vi "Chamber control Feb_2018.vi"() -> ()   [LabVIEW 2014]
doc: "This template is for the Queued Message Handler design pattern.\n\nThe Event Handling Loop generates messages based on user interface actions.\n\nThe Message Handling Loop processes messages generated by the Event Handling Loop, or by other messages. The messages are string values, so new messages can be added easily to the Message Cases case structure in the Message Handling Loop. Each message cluster can also provide an optional value for Message Data, which is a variant that can be converted to whatever message-specific data is required."
uses:
  <vilib>/Analysis/baseanly.llb/Mean (DBL).vi
  <vilib>/Instr/_visa.llb/VISA Configure Serial Port (Instr).vi
  Environmental Chamber LabVIEW and Instruments/Drivers and Software/Keithley 2100 Series/Public/Configure/Configure 2 Wire Resistance.vi
  <vilib>/Utility/file.llb/Write To Spreadsheet File (string).vi
  <vilib>/Utility/file.llb/Read From Spreadsheet File (string).vi
  Environmental Chamber LabVIEW and Instruments/Drivers and Software/LabVIEW 8.2 Drivers/keithley_24xx/Keithley 24XX/Public/Data/Read (Single Point).vi
  Environmental Chamber LabVIEW and Instruments/Drivers and Software/keithley_6430/Keithley 6430/Public/Data/Read (Single Point).vi
  Environmental Chamber LabVIEW and Instruments/Drivers and Software/keithley_6430/Keithley 6430/Keithley 6430.lvlib
  Environmental Chamber LabVIEW and Instruments/Drivers and Software/Keithley 2100 Series/Keithley 2100 Series.lvlib
  Environmental Chamber LabVIEW and Instruments/Drivers and Software/keithley_24xx/Keithley 24XX/Keithley 24XX.lvlib
  <vilib>/Analysis/NI_AALBase.lvlib
panel:
  in  "K2420 Applied Voltage (V)":dbl=0.05
  in  "SYSTEM CONTROL":T1={"valve % open"=0.0, "Desired pressure"=0.0, "set Vapor sccm"=0.0, "set Gas sccm"=0.0, "Valve mode"=enum."% Open", "Pressure Mode"=enum."Abs. pressure", "analyte partial pressure"=23.8, "Actual"=0.0, "Read pressure (Torr)"=0.0, "Read vapor flow (sccm)"=0.0, "Read gas flow (sccm)"=0.0, "Save now"=FALSE, "Stop after seq."=TRUE, "Turbo pump\nauto on"=TRUE, "Integrate points"=0} caption="Pressure settings" {"Integrate points" min=0 max=100 step=1; "analyte partial pressure" min=0.0 max=100.0 step=5.0; "set Gas sccm" min=0 max=200 step=5; "set Vapor sccm" min=0 max=200 step=5; "Desired pressure" min=0.0 max=760.0 step=5.0; "valve % open" min=0.0 max=100.0 step=5.0 format="%#_2f"}
  in  "SAVE SAMPLE / ANALYTE NAMES":T2={"QCM1"="", "QCM2"="", "QCM3"="", "QCM4"="broken", "QCM5"="NOT WORKING", "QCM6"="", "SRS"="bareAu", "K-2420"="", "K-6430"="", "K-2100"="", "Gas"="NOT WORKING", "Vapor"="H2O", "Notes"=""} caption="Save samplffe names"
  in  "Clear all charts":bool
  out "K-6430":dbl(graph)
  out "K-2420":dbl(graph)
  out "File":path caption="DATA FILE"
  in  "Stop":bool
  out "QCM plot":T3(graph)
  out "K-2100":dbl(graph)
  out "State date/time":string caption="Program start time"
  out "J-KEM temp":dbl(graph)
  out "saving data?":bool
  out "pressure chart":dbl(graph)
  out "arduino qcm stack plot":T4(graph)
  in  "SEQUENCE":T5 {"preview" items=["pressure", "gas flow", "vapor flow", "bias"]}
  # "100"
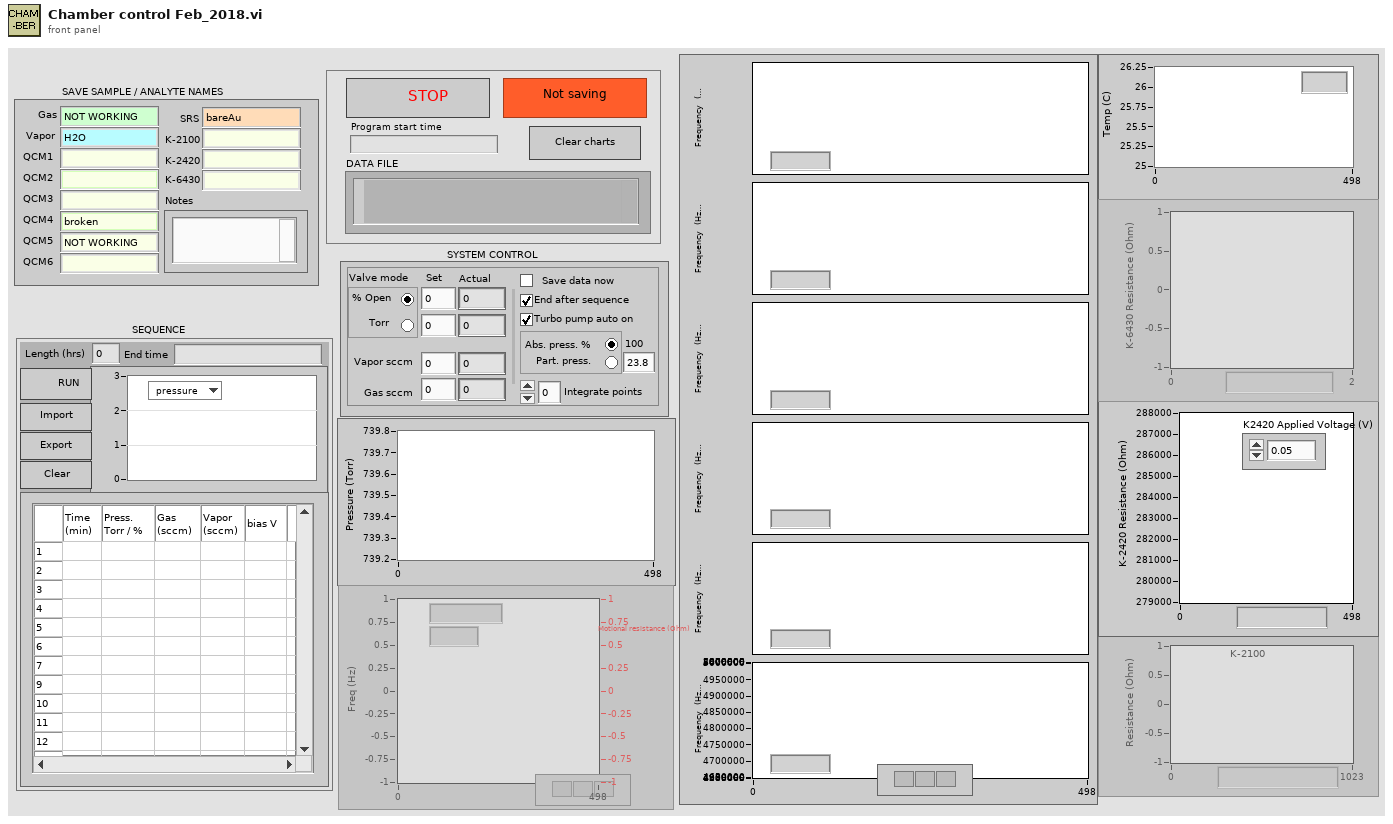
[diagram p1: front panel]
types:
  T1 = cluster{"valve % open":dbl, "Desired pressure":dbl, "set Vapor sccm":sgl, "set Gas sccm":sgl, "Valve mode":enum32{"% Open", "Torr "}, "Pressure Mode":enum32{"Abs. pressure", " Part. pressure"}, "analyte partial pressure":dbl, "Actual":dbl, "Read pressure (Torr)":dbl, "Read vapor flow (sccm)":dbl, "Read gas flow (sccm)":dbl, "Save now":bool, "Stop after seq.":bool, "Turbo pump\nauto on":bool, "Integrate points":i32}
  T2 = cluster{"QCM1":string, "QCM2":string, "QCM3":string, "QCM4":string, "QCM5":string, "QCM6":string, "SRS":string, "K-2420":string, "K-6430":string, "K-2100":string, "Gas":string, "Vapor":string, "Notes":string}
  T3 = cluster{"Frequency out":dbl, "Resistance out":dbl}
  T4 = cluster{"[0]":dbl, "[1]":dbl, "[2]":dbl, "[3]":dbl, "[4]":dbl, "[5]":dbl}
  T5 = cluster{"Run Sequence":bool, "User-defined\nsequence":string[][], "preview":u16, "Sequence\npreview":cluster{dbl[], dbl[]}[], "Save sequence":bool, "Clear sequence":bool, "Import sequence file":bool, "Length (hrs)":dbl, "End time":string}
  T6 = cluster{"Keithley 6430":bool, "J-KEM":bool, "Keithley 2420":bool, "Keithley 2100":bool, "SRS QCM":bool, "Pressure control":bool, "Arduino":bool}
  T7 = enum16{"open", "replace", "create", "open or create", "replace or create", "replace or create with confirmation"}
  T8 = cluster{"Arduino 1":refnum<visa-resource-name>, "Arduino 2":refnum<visa-resource-name>, "Arduino 3":refnum<visa-resource-name>, "Arduino 4":refnum<visa-resource-name>, "Arduino 5":refnum<visa-resource-name>, "Arduino 6":refnum<visa-resource-name>}
  T9 = enum8{"Enabled", "Disabled", "Disabled and Grayed Out"}
  T10 = cluster{"[0]":dbl, "[1]":dbl, "[2]":dbl, "[3]":dbl, "[4]":dbl, "[5]":dbl}[]
  T11 = cluster{"Frequency out":dbl, "Resistance out":dbl}[]
  T12 = cluster{"VISA resource name":refnum<visa-resource-name>, "error out":errorcluster, bool}
  T13 = cluster{"VISA resource name out":refnum<visa-resource-name>, "error out":errorcluster, bool}
  T14 = cluster{bool, "task out":refnum<k21>, "error out":errorcluster, "task out":refnum<k21>, "error out":errorcluster, "turbo pump":refnum<visa-resource-name>, "error out":errorcluster}
  T15 = cluster{bool, "task out":refnum<k21>, "error out":errorcluster, "task out":refnum<k21>, "error out":errorcluster, "VISA resource name out":refnum<visa-resource-name>, "error out":errorcluster}
  T16 = cluster{bool, "VISA resource name":refnum<visa-resource-name>, "error out":errorcluster}
  T17 = cluster{bool, "VISA resource name out":refnum<visa-resource-name>, "error out":errorcluster}
  T18 = cluster{bool, "VISA in":refnum<visa-resource-name>, "error out":errorcluster}
  T19 = cluster{bool, "VISA out":refnum<visa-resource-name>, "error out":errorcluster}
  T20 = cluster{"Arduino address":refnum<visa-resource-name>, "error in (no error)":errorcluster, "Arduino address 2":refnum<visa-resource-name>, "error in (no error) 2":errorcluster, "Arduino address 3":refnum<visa-resource-name>, "error in (no error) 3":errorcluster, "Arduino address 4":refnum<visa-resource-name>, "error in (no error) 4":errorcluster, "Arduino address 5":refnum<visa-resource-name>, "error in (no error) 5":errorcluster, "Arduino address 6":refnum<visa-resource-name>, "error in (no error) 6":errorcluster, "arduinos on?":bool}
  T21 = cluster{string[][], path, "data headers":string[]}
  T22 = cluster{"valve % open":dbl, "Desired pressure":dbl, "set Vapor sccm":sgl, "set Gas sccm":sgl, "Valve mode":enum32{"% Open", "Torr "}, "Pressure Mode":enum32{"Abs. pressure", " Part. pressure"}, "analyte partial pressure":dbl}
  T23 = cluster{"Boolean":bool, "VISA resource name out":refnum<visa-resource-name>, "error out":errorcluster}
  T24 = cluster{"Boolean":bool, "VISA out":refnum<visa-resource-name>, "error out":errorcluster}
  T25 = cluster{"Boolean":bool, "Arduino address":refnum<visa-resource-name>, "error in (no error)":errorcluster, "Arduino address 2":refnum<visa-resource-name>, "error in (no error) 2":errorcluster, "Arduino address 3":refnum<visa-resource-name>, "error in (no error) 3":errorcluster, "Arduino address 4":refnum<visa-resource-name>, "error in (no error) 4":errorcluster, "Arduino address 5":refnum<visa-resource-name>, "error in (no error) 5":errorcluster, "Arduino address 6":refnum<visa-resource-name>, "error in (no error) 6":errorcluster}
  T26 = cluster{"arduino addresses out":cluster{"Boolean":bool, "Arduino address":refnum<visa-resource-name>, "error in (no error)":errorcluster, "Arduino address 2":refnum<visa-resource-name>, "error in (no error) 2":errorcluster, "Arduino address 3":refnum<visa-resource-name>, "error in (no error) 3":errorcluster, "Arduino address 4":refnum<visa-resource-name>, "error in (no error) 4":errorcluster, "Arduino address 5":refnum<visa-resource-name>, "error in (no error) 5":errorcluster, "Arduino address 6":refnum<visa-resource-name>, "error in (no error) 6":errorcluster}, cluster{bool, "VISA resource name out":refnum<visa-resource-name>, "error out":errorcluster}, "Address out":cluster{"Boolean":bool, "VISA resource name out":refnum<visa-resource-name>, "error out":errorcluster}, cluster{bool, "VISA resource name out":refnum<visa-resource-name>, "error out":errorcluster}, cluster{bool, "VISA resource name out":refnum<visa-resource-name>, "error out":errorcluster}, "SRS address out":cluster{"Boolean":bool, "VISA out":refnum<visa-resource-name>, "error out":errorcluster}}
  T27 = cluster{"User-defined\nsequence":string[][], "Present (s)":dbl, "current  step # in":i32, "sequence end time in":timestamp}
  T28 = cluster{"current  step # in":i32, "sequence end time in":timestamp, "Boolean":bool}
  T29 = cluster{"press/RH/gas/vapor":cluster{"pressure":string, "RH":string, "gas flow":string, "vapor flow":string}, "Cluster":cluster{"Valve position (%)":dbl, "read pressure":dbl, "read vapor flow":dbl, "read gas flow":dbl}}
  T30 = cluster{"Boolean":bool, "task out":refnum<k21>, "error out":errorcluster, "task out":refnum<k21>, "error out":errorcluster, "VISA resource name out":refnum<visa-resource-name>, "error out":errorcluster}
  T31 = cluster{"pressure":string, "RH":string, "gas flow":string, "vapor flow":string}
  T32 = cluster{"Valve position (%)":dbl, "read pressure":dbl, "read vapor flow":dbl, "read gas flow":dbl}
  T33 = cluster{"[0]":string, "[1]":string, "[2]":string, "[3]":string, "[4]":string, "[5]":string}
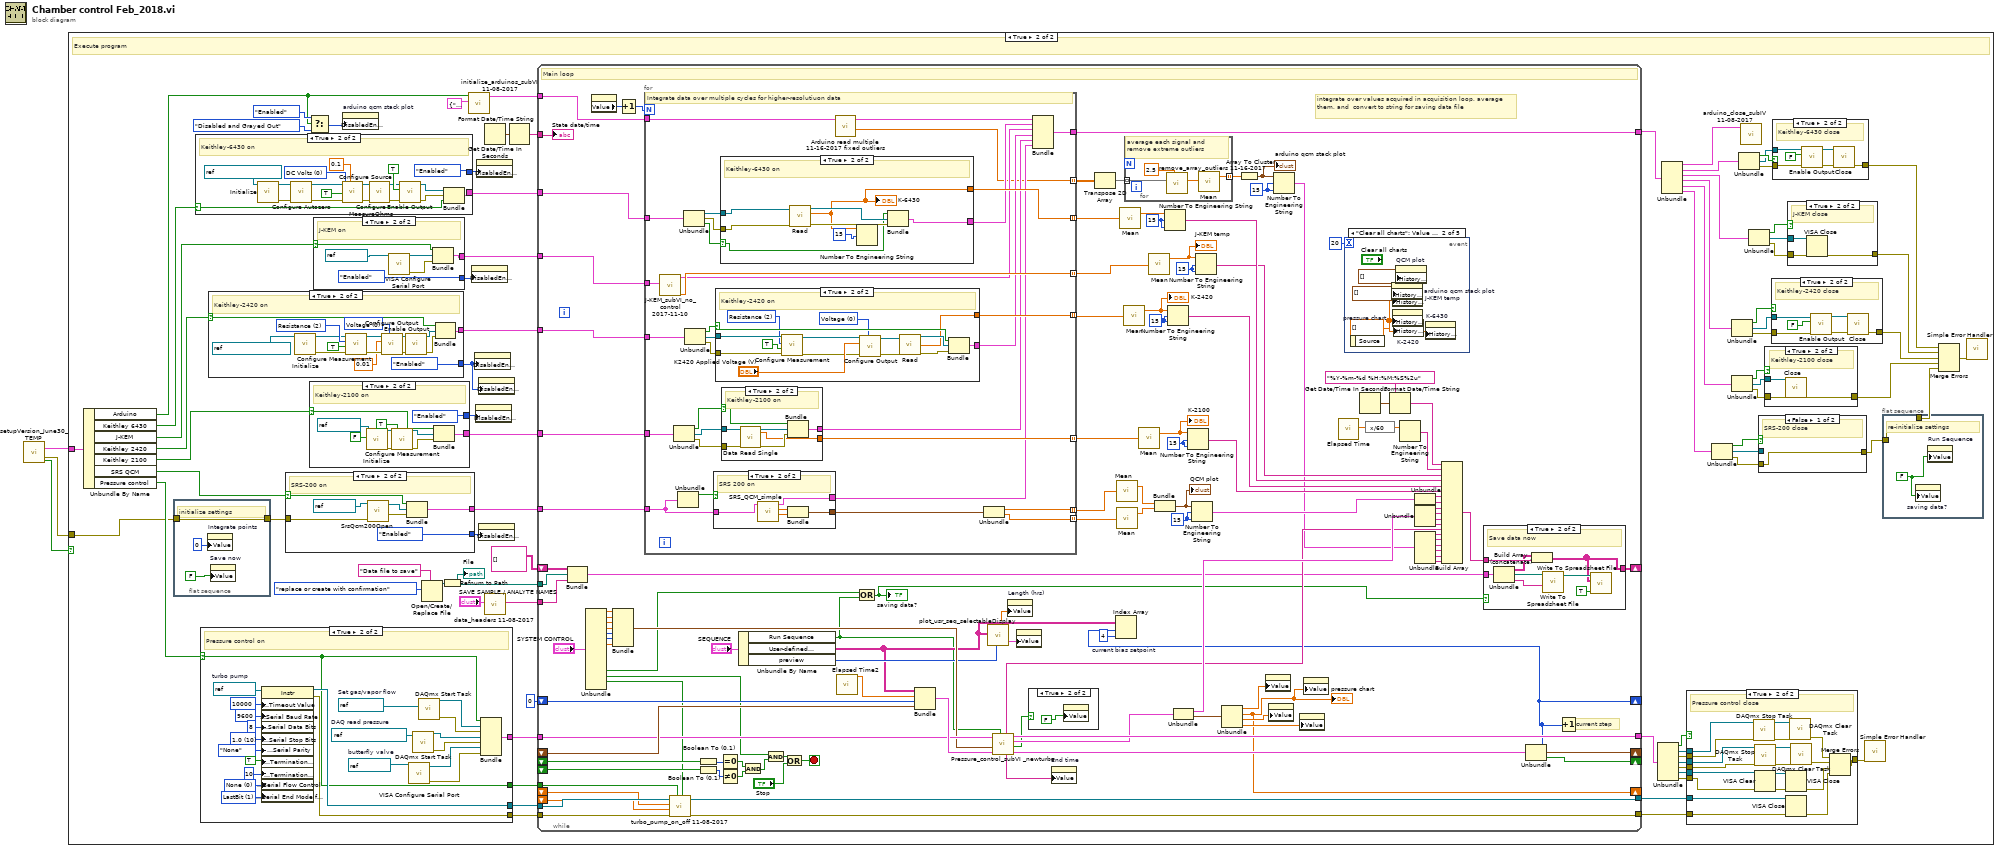
[diagram p0: block diagram]
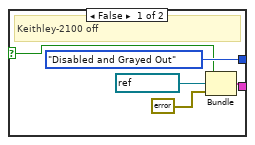
[diagram p4: hidden frame]
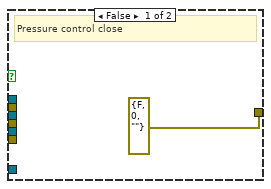
[diagram p5: hidden frame]
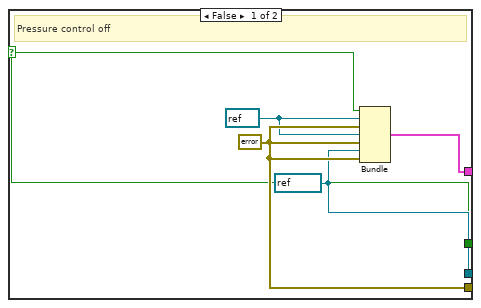
[diagram p6: hidden frame]
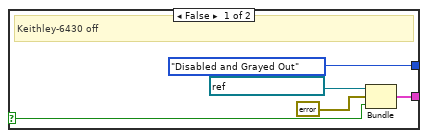
[diagram p8: hidden frame]
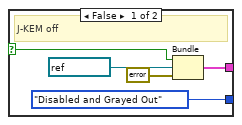
[diagram p10: hidden frame]
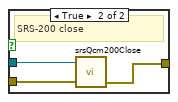
[diagram p11: hidden frame]
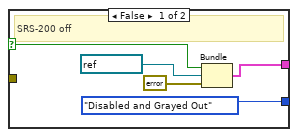
[diagram p12: hidden frame]
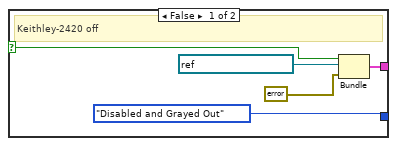
[diagram p14: hidden frame]
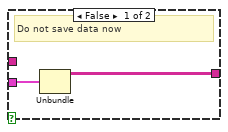
[diagram p15: hidden frame]
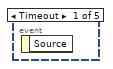
[diagram p16: hidden frame]
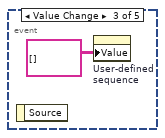
[diagram p17: hidden frame]
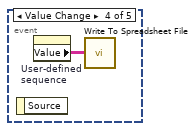
[diagram p18: hidden frame]
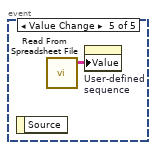
[diagram p19: hidden frame]
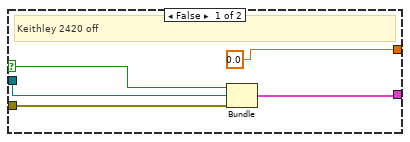
[diagram p20: hidden frame]
diagram:
  n1 = call "setupVersion_June30_TEMP.vi"() -> ("Instruments on/off"=w1:T6, "error IO"=w2:errorcluster, "OK"=w3:bool)  [unwired: 13 in]
  n2 = case shown="True" w3 {
    tunnel: w2 -> [_ w47]
    tunnel: w1 -> [_ w54]
    frame False {
      # "Cancel program"
    }
    frame True {
      # "Execute program"
      n3 = Unbundle By Name(w54) -> ("Arduino"=w26:bool, "Keithley 6430"=w53:bool, "J-KEM"=w52:bool, "Keithley 2420"=w51:bool, "Keithley 2100"=w50:bool, "SRS QCM"=w49:bool, "Pressure control"=w48:bool)
      n4 = flat-sequence {
        tunnel: [w85] -> w46
        tunnel: w47 -> [w85]
        frame #0 {
          # "initialize settings"
          n5 = property on="Integrate points" class="DigNum (strict)"("Value"=0) -> ()  [unwired: 2 in, 2 out]
          n6 = property on="Save now" class="Bool (strict)"("Value"=FALSE) -> ()  [unwired: 2 in, 2 out]
        }
      }
      n7 = case shown="True" w53 {
        selector: w53 -> [w163 w183]
        tunnel: [T9."Disabled and Grayed Out" ("Disabled") T9."Enabled" ("Disabled")] -> w32
        tunnel: [w162 w182] -> w30
        frame False {
          # "Keithley-6430 off"
          n8 = Bundle("VISA resource name"=refnum<visa-resource-name> "GPIB0::29::INSTR", "error out"=errorcluster {"status"=FALSE, "code"=0, "source"=""}, w163) -> (w162:T12)  [unwired: 1 in]
        }
        frame True {
          w170 = u16 0 items=["DC Volts", "DC Current"] ("Source Function (0: DC Volts)")
          # "Keithley-6430 on"
          n9 = call "Initialize.vi"("VISA resource name"=refnum<visa-resource-name> "GPIB2::19::INSTR") -> ("error out"=w176:errorcluster, "VISA resource name out"=w177:refnum<visa-resource-name>)  [unwired: 4 in, 5 out]
          n10 = call "Configure Autozero.vi"("error in (no error)"=w176, "VISA resource name"=w177) -> ("error out"=w173:errorcluster, "VISA resource name out"=w175:refnum<visa-resource-name>)  [unwired: 8 in]
          n11 = call "Configure Source.vi"("V-Source Level [V]"=0.1, "error in (no error)"=w173, "Auto Range (T:Enable)"=TRUE, "Source Function (0: DC Volts)"=w170, "VISA resource name"=w175) -> ("error out"=w172:errorcluster, "VISA resource name out"=w174:refnum<visa-resource-name>)  [unwired: 5 in]
          n12 = call "Configure MeasureOhms.vi"("error in (no error)"=w172, "VISA resource name"=w174) -> ("error out"=w181:errorcluster, "VISA resource name out"=w179:refnum<visa-resource-name>)  [unwired: 4 in, 4 out]
          n13 = call "Enable Output.vi"("error in (no error)"=w181, "Enable Output (F:Off)"=TRUE ("Output (F:Off)"), "VISA resource name"=w179) -> ("error out"=w168:errorcluster, "VISA resource name out"=w169:refnum<visa-resource-name>)  [unwired: 7 out]
          n14 = Bundle("VISA resource name out"=w169, "error out"=w168, w183) -> (w182:T13)  [unwired: 1 in]
        }
      }
      n15 = case shown="True" w48 {
        selector: w48 -> [w127 w133]
        tunnel: [w131 w134] -> w45
        tunnel: [w130 w132] -> w37
        tunnel: [w128 w135] -> w38
        tunnel: [w127 w133] -> w36
        frame False {
          w128 = refnum<visa-resource-name> refnum ("turbo pump")
          w129 = refnum<k21> refnum ("task out")
          w130 = errorcluster {"status"=FALSE, "code"=0, "source"=""} ("error out")
          # "Pressure control off"
          n16 = Bundle(w127, "task out"=w129, "error out"=w130, "task out"=w129, "error out"=w130, "turbo pump"=w128, "error out"=w130) -> (w131:T14)  [unwired: 1 in]
        }
        frame True {
          w139 = u16 1 items=["None", "LastBit", "TermChar"] ("Serial Settings:Serial End Mode for Reads")
          w137 = u16 0 items=["None", "XON/XOFF", "RTS/CTS", "XON/XOFF & RTS/CTS", "DTR/DSR", "XON/XOFF & DTR/DSR"] ("flow control (0:none)")
          w140 = u16 10 items=["1.0"=10, "1.5"=15, "2.0"=20] ("stop bits (10: 1 bit)")
          w136 = refnum<visa-resource-name> "COM7"  # turbo pump
          w152 = refnum<visa-resource-name> "COM5"  # butterfly valve
          w153 = refnum<k21> "Setflow"  # Set gas/vapor flow
          w154 = refnum<k21> "AllDaqReadings"  # DAQ read pressure
          # "Pressure control on"
          n17 = property class="Instr"(reference=w136, "General Settings:Timeout Value"=u32 10000 ("timeout (10sec)"), "Serial Settings:Serial Baud Rate"=u32 9600 ("baud rate (9600)"), "Serial Settings:Serial Data Bits"=u16 8 ("data bits (8)"), "Serial Settings:Serial Stop Bits"=w140, "Serial Settings:Serial Parity"=enum16{"None", "Odd", "Even", "Mark", "Space"}."None" ("parity (0:none)"), "Message Based Settings:Termination Character Enable"=TRUE ("Enable Termination\nChar (T)"), "Message Based Settings:Termination Character"=u8 10 ("termination char\n(0xA = '\\n' = LF)"), "Serial Settings:Serial Flow Control"=w137, "Serial Settings:Serial End Mode for Reads"=w139) -> (reference out=w135:refnum<visa-resource-name>, error out=w132:errorcluster)  [unwired: 1 in]
          n18 = call-poly "VISA Configure Serial Port"("VISA resource name"=w152) -> ("VISA resource name out"=w147:refnum<visa-resource-name>, "error out"=w146:errorcluster)  [unwired: 13 in]
          n19 = call <vilib>:"DAQmx Start Task.vi"("task/channels in"=w154) -> ("task out"=w149:refnum<k21>, "error out"=w148:errorcluster)  [unwired: 13 in]
          n20 = call <vilib>:"DAQmx Start Task.vi"("task/channels in"=w153) -> ("task out"=w151:refnum<k21>, "error out"=w150:errorcluster)  [unwired: 13 in]
          n21 = Bundle(w133, "task out"=w151, "error out"=w150, "task out"=w149, "error out"=w148, "VISA resource name out"=w147, "error out"=w146) -> (w134:T15)  [unwired: 1 in]
        }
      }
      n22 = case shown="True" w51 {
        selector: w51 -> [w226 w231]
        tunnel: [T9."Disabled and Grayed Out" ("Disabled") T9."Enabled" ("Disabled")] -> w11
        tunnel: [w224 w228] -> w29
        frame False {
          # "Keithley-2420 off"
          n23 = Bundle(w226, "VISA resource name"=refnum<visa-resource-name> "GPIB1::24::INSTR", "error out"=errorcluster {"status"=FALSE, "code"=0, "source"=""}) -> (w224:T16)  [unwired: 1 in]
        }
        frame True {
          w237 = u16 0 items=["Voltage", "Current"] ("Source Mode  (0: Voltage)")
          w242 = u16 2 items=["Volts", "Current", "Resistance"] ("Function (0: Volts)")
          # "Keithley-2420 on"
          n24 = call "Initialize.vi"("VISA resource name"=refnum<visa-resource-name> "GPIB1::24::INSTR") -> ("error out"=w232:errorcluster, "VISA resource name out"=w233:refnum<visa-resource-name>)  [unwired: 9 in]
          n25 = call "Configure Measurement.vi"("error in (no error)"=w232, "Enable Auto Range (T:Enable)"=TRUE, "Function (0: Volts)"=w242, "VISA resource name"=w233) -> ("error out"=w241:errorcluster, "VISA resource name out"=w240:refnum<visa-resource-name>)  [unwired: 6 in]
          n26 = call "Configure Output.vi"("Source Mode  (0: Voltage)"=w237, "error in (no error)"=w241, "Output Level (0)"=0.01 ("K2420 Applied Voltage (V) 2"), "VISA resource name"=w240) -> ("error out"=w239:errorcluster, "VISA resource name out"=w238:refnum<visa-resource-name>)  [unwired: 6 in]
          n27 = call "Enable Output.vi"("error in (no error)"=w239, "VISA resource name"=w238) -> ("error out"=w229:errorcluster, "VISA resource name out"=w230:refnum<visa-resource-name>)  [unwired: 8 in]
          n28 = Bundle(w231, "VISA resource name out"=w230, "error out"=w229) -> (w228:T17)  [unwired: 1 in]
        }
      }
      n29 = case shown="True" w49 {
        selector: w49 -> [w205 w211]
        tunnel: w46 -> [_ w214]
        tunnel: [T9."Disabled and Grayed Out" ("Disabled") T9."Enabled" ("Disabled")] -> w66
        tunnel: [w204 w210] -> w27
        frame False {
          # "SRS-200 off"
          n30 = Bundle(w205, "VISA in"=refnum<visa-resource-name> "COM6", "error out"=errorcluster {"status"=FALSE, "code"=0, "source"=""}) -> (w204:T18)  [unwired: 1 in]
        }
        frame True {
          # "SRS-200 on"
          n31 = call "SrsQcm200Open.vi"("error in"=w214, "VISA in"=refnum<visa-resource-name> "COM6") -> ("error out"=w209:errorcluster, "VISA out"=w212:refnum<visa-resource-name>)  [unwired: 3 in]
          n32 = Bundle(w211, "VISA out"=w212, "error out"=w209) -> (w210:T19)  [unwired: 1 in]
        }
      }
      n33 = Select(t=T9."Enabled" ("Disabled"), s=w26, f=T9."Disabled and Grayed Out" ("Disabled")) -> (s? t:f=w33:T9)
      n34 = case shown="True" w50 {
        selector: w50 -> [w95 w99]
        tunnel: [T9."Disabled and Grayed Out" ("Disabled") T9."Enabled" ("Disabled")] -> w63
        tunnel: [w92 w100] -> w28
        frame False {
          # "Keithley-2100 off"
          n35 = Bundle(w95, "VISA resource name out"=refnum<visa-resource-name> "K-2100", "error out"=errorcluster {"status"=FALSE, "code"=0, "source"=""}) -> (w92:T17)  [unwired: 1 in]
        }
        frame True {
          # "Keithley-2100 on"
          n36 = call "Initialize.vi"("VISA resource name"=refnum<visa-resource-name> "K-2100", "Reset? (T: Reset)"=FALSE) -> ("VISA resource name out"=w104:refnum<visa-resource-name>, "error out"=w103:errorcluster)  [unwired: 16 in]
          n37 = call-poly "Configure Measurement.vi"("VISA resource name"=w104, "error in (no error)"=w103, "Auto Range? (T: Auto)"=TRUE) -> ("VISA resource name out"=w98:refnum<visa-resource-name>, "error out"=w97:errorcluster)  [unwired: 15 in]
          n38 = Bundle(w99, "VISA resource name out"=w98, "error out"=w97) -> (w100:T17)  [unwired: 1 in]
        }
      }
      n39 = case shown="True" w52 {
        selector: w52 -> [w190 w196]
        tunnel: [w191 w197] -> w75
        tunnel: [T9."Disabled and Grayed Out" ("Disabled") T9."Enabled" ("Disabled")] -> w31
        frame False {
          # "J-KEM off"
          n40 = Bundle(w190, "VISA resource name"=refnum<visa-resource-name> "COM3", "error out"=errorcluster {"status"=FALSE, "code"=0, "source"=""}) -> (w191:T16)  [unwired: 1 in]
        }
        frame True {
          # "J-KEM on"
          n41 = call-poly "VISA Configure Serial Port"("VISA resource name"=refnum<visa-resource-name> "COM3") -> ("VISA resource name out"=w198:refnum<visa-resource-name>, "error out"=w195:errorcluster)  [unwired: 13 in]
          n42 = Bundle(w196, "VISA resource name out"=w198, "error out"=w195) -> (w197:T17)  [unwired: 1 in]
        }
      }
      n43 = property on="arduino qcm stack plot" class="WFChart (strict)"("DisabledEnum"=w33) -> ()  [unwired: 2 in, 2 out]
      n44 = Open/Create/Replace File(prompt="Data file to save", operation (0:open)=T7."replace or create with confirmation") -> (refnum out=w9:refnum<file>)  [unwired: 4 in, 2 out]
      n45 = Refnum to Path(1:w9) -> (0:w5:path)
      "File" <- w5
      n46 = call "initialize_arduinos_subVI 11-08-2017.vi"("arduino 1-6 addresses"=T8 {"Arduino 1"="COM25", "Arduino 2"="COM48", "Arduino 3"="COM21", "Arduino 4"="COM22", "Arduino 5"="COM23", "Arduino 6"="COM24"} ("Arduino COMs"), "arduinos on?"=w26) -> ("arduino addresses out"=w65:T20)  [unwired: 9 in]
      n47 = property on="J-KEM temp" class="WFChart (strict)"("DisabledEnum"=w31) -> ()  [unwired: 2 in, 2 out]
      n48 = property on="K-2420" class="WFChart (strict)"("DisabledEnum"=w11) -> ()  [unwired: 2 in, 2 out]
      n49 = property on="K-2100" class="WFChart (strict)"("DisabledEnum"=w63) -> ()  [unwired: 2 in, 2 out]
      n50 = property on="K-6430" class="WFChart (strict)"("DisabledEnum"=w32) -> ()  [unwired: 2 in, 2 out]
      n51 = property on="K2420 Applied Voltage (V)" class="DigNum (strict)"("DisabledEnum"=w11) -> ()  [unwired: 2 in, 2 out]
      n52 = property on="QCM plot" class="WFChart (strict)"("DisabledEnum"=w66) -> ()  [unwired: 2 in, 2 out]
      n53 = call "data_headers 11-08-2017.vi"("Sample names"="SAVE SAMPLE / ANALYTE NAMES") -> ("data headers"=w4:string[])  [unwired: 10 in]
      n54 = Get Date/Time In Seconds() -> (seconds since 1Jan1904=w12:timestamp)
      n55 = Format Date/Time String(seconds (now)=w12) -> (date/time string=w62:string)  [unwired: 2 in]
      n56 = while {
        tunnel: w75 -> [w363]
        tunnel: w5 -> [w250]
        tunnel: w65 -> [w316]
        tunnel: w62 -> [w345]
        tunnel: w45 -> [w332]
        shift-right: [w312] -> _
        shift-left: 0 ("1st step") -> [w337]
        shift-right: [w342] -> _
        shift-left: _ -> [w340]
        shift-right: [w341] -> _
        shift-left: _ -> [w339]
        shift-left: _ -> [w338]
        tunnel: [w336] -> w58
        tunnel: w38 -> [w331]
        tunnel: w37 -> [w330]
        tunnel: w36 -> [w315]
        tunnel: [w328] -> w35
        tunnel: [w329] -> w34
        tunnel: w30 -> [w320]
        tunnel: w29 -> [w319]
        tunnel: w28 -> [w318]
        tunnel: w27 -> [w317]
        shift-right: [w256] -> _
        shift-left: _ -> [w314]
        shift-left: _ -> [w313]
        tunnel: [w288] -> w19
        shift-right: [w253] -> _
        shift-left: string[][] [] -> [w251]
        tunnel: w4 -> [w249]
        stop <- w351 stop-if-true
        w280 = i16 15 ("width (-)")
        w281 = i16 15 ("width (-)")
        w282 = i16 15 ("width (-)")
        w283 = i16 15 ("width (-)")
        w284 = i16 15 ("width (-)")
        w285 = i16 15 ("width (-)")
        # "current step"
        # "integrate over values acquired in acquisition loop, average them, and  convert to string for saving data file"
        # "Main loop"
        n57 = Bundle(w251, w250, "data headers"=w249) -> (w248:T21)  [unwired: 1 in]
        n58 = Unbundle("SYSTEM CONTROL") -> ("valve % open"=w273:dbl, "Desired pressure"=w272:dbl, "set Vapor sccm"=w271:sgl, "set Gas sccm"=w270:sgl, "Valve mode"=w269:enum32{"% Open", "Torr "}, "Pressure Mode"=w268:enum32{"Abs. pressure", " Part. pressure"}, "analyte partial pressure"=w267:dbl, "Save now"=w259:bool, "Stop after seq."=w258:bool, "Turbo pump\nauto on"=w257:bool)  [unwired: 5 out]
        n59 = property on="Integrate points" class="DigNum (strict)"() -> ("Value"=w245:i32)  [unwired: 2 in, 2 out]
        n60 = Bundle("valve % open"=w273, "Desired pressure"=w272, "set Vapor sccm"=w271, "set Gas sccm"=w270, "Valve mode"=w269, "Pressure Mode"=w268, "analyte partial pressure"=w267) -> (w274:T22)  [unwired: 1 in]
        n61 = Increment(x=w245) -> (x+1=w287:i32)
        n62 = for {
          N: w287 -> [_]
          tunnel: w320 -> [w414]
          tunnel: w319 -> [w411]
          tunnel: w318 -> [w407]
          tunnel: w317 -> [w388]
          tunnel: w316 -> [w387]
          tunnel: w363 -> [w415]
          tunnel: [w402] -> w307 mode=indexing
          tunnel: [w401] -> w302 mode=indexing
          tunnel: [w400] -> w305 mode=indexing
          tunnel: [w399] -> w301 mode=indexing
          tunnel: [w397] -> w299 mode=indexing
          tunnel: [w396] -> w298 mode=indexing
          tunnel: [w386] -> w293 mode=indexing
          tunnel: [w390] -> w288
          # "Integrate data over multiple cycles for higher-resolutiuon data"
          n63 = call "J-KEM_subVI_no_control 2017-11-10.vi"("Address in"=w415) -> ("Temp (C)"=w400:dbl, "Address out"=w394:T23)  [unwired: 9 in]
          n64 = Unbundle(w407) -> (w406:bool, "VISA resource name out"=w405:refnum<visa-resource-name>, "error out"=w404:errorcluster)
          n65 = Unbundle(w388) -> (w389:bool)  [unwired: 2 out]
          n66 = Unbundle(w414) -> ("VISA resource name out"=w413:refnum<visa-resource-name>, "error out"=w403:errorcluster, w412:bool)
          n67 = Unbundle(w411) -> (w410:bool, "VISA resource name out"=w409:refnum<visa-resource-name>, "error out"=w408:errorcluster)
          n68 = case "SRS QCM" shown="True" w389 {
            tunnel: [w461 w467] -> w391
            tunnel: [T3 {"Frequency out"=0.0, "Resistance out"=0.0} ("freq, MR") w464] -> w398
            tunnel: w388 -> [w461 w463]
            frame False {
              # "SRS QCM off"
            }
            frame True {
              # "SRS 200 on"
              n69 = call "SRS_QCM_simple.vi"("SRS address in"=w463) -> ("Resistance out"=w466:dbl, "Frequency out"=w465:dbl, "SRS address out"=w467:T24)  [unwired: 8 in]
              n70 = Bundle("Frequency out"=w465, "Resistance out"=w466) -> (w464:T3)  [unwired: 1 in]
            }
          }
          n71 = case shown="True" w410 {
            selector: w410 -> [w420 w435]
            tunnel: [w417 w434] -> w393
            tunnel: w409 -> [w419 w427]
            tunnel: w408 -> [w418 w425]
            tunnel: [sgl 0.0 ("Resistance") w422] -> w401
            frame False {
              # "Keithley 2420 off"
              n72 = Bundle(w420, "VISA resource name out"=w419, "error out"=w418) -> (w417:T17)  [unwired: 1 in]
            }
            frame True {
              w423 = u16 2 items=["Volts", "Current", "Resistance"] ("Function (0: Volts)")
              w431 = u16 0 items=["Voltage", "Current"] ("Source Mode  (0: Voltage)")
              # "Keithley-2420 on"
              n73 = call "Configure Measurement.vi"("error in (no error)"=w425, "Enable Auto Range (T:Enable)"=TRUE, "Function (0: Volts)"=w423, "VISA resource name"=w427) -> ("error out"=w424:errorcluster, "VISA resource name out"=w426:refnum<visa-resource-name>)  [unwired: 6 in]
              n74 = call "Configure Output.vi"("Source Mode  (0: Voltage)"=w431, "error in (no error)"=w424, "Output Level (0)"="K2420 Applied Voltage (V)", "VISA resource name"=w426) -> ("error out"=w429:errorcluster, "VISA resource name out"=w430:refnum<visa-resource-name>)  [unwired: 6 in]
              n75 = call-poly "Read.vi"("VISA resource name"=w430, "error in (no error)"=w429) -> ("VISA resource name out"=w433:refnum<visa-resource-name>, "Resistance"=w422:sgl, "error out"=w432:errorcluster)  [unwired: 7 in, 4 out]
              n76 = Bundle(w435, "VISA resource name out"=w433, "error out"=w432) -> (w434:T17)  [unwired: 1 in]
            }
          }
          n77 = case "Keithley 6430" shown="True" w412 {
            selector: w412 -> [w452 w455]
            tunnel: w413 -> [w451 w457]
            tunnel: [w450 w454] -> w395
            tunnel: w403 -> [w449 w456]
            tunnel: [0.0 ("K6340 Bias (V)") w453] -> w402
            frame False {
              # "Keithley-6430 off"
              n78 = Bundle(w452, "VISA resource name out"=w451, "error out"=w449) -> (w450:T17)  [unwired: 1 in]
            }
            frame True {
              # "Keithley-6430 on"
              n79 = call-poly "Read.vi"("error in (no error)"=w456, "VISA resource name"=w457) -> ("error out"=w458:errorcluster, "Measurement"=w453:dbl, "VISA resource name out"=w459:refnum<visa-resource-name>)  [unwired: 1 in, 6 out]
              "K-6430" <- w453
              n80 = Number To Engineering String(3:i16 15 ("width (-)"), 4:w453) -> ()  [unwired: 2 in, 1 out]
              n81 = Bundle(w455, "VISA resource name out"=w459, "error out"=w458) -> (w454:T17)  [unwired: 1 in]
            }
          }
          n82 = case shown="True" w406 {
            selector: w406 -> [w440 w445]
            tunnel: w405 -> [w438 w447]
            tunnel: w404 -> [w439 w446]
            tunnel: [w437 w442] -> w392
            tunnel: [0.0 ("Measurement") w441] -> w399
            frame False {
              # "Keithley-2100 off"
              n83 = Bundle(w440, "VISA resource name out"=w438, "error out"=w439) -> (w437:T17)  [unwired: 1 in]
            }
            frame True {
              # "Keithley-2100 on"
              n84 = call "Data Read Single.vi"("VISA resource name"=w447, "error in (no error)"=w446) -> ("VISA resource name out"=w444:refnum<visa-resource-name>, "Measurement"=w441:dbl, "error out"=w443:errorcluster)  [unwired: 15 in]
              n85 = Bundle(w445, "VISA resource name out"=w444, "error out"=w443) -> (w442:T17)  [unwired: 1 in]
            }
          }
          n86 = call "Arduino read multiple 11-16-2017 fixed outliers.vi"("arduino addresses in"=w387) -> ("freq out"=w386:dbl[], "arduino addresses out"=w385:T25)  [unwired: 8 in]
          n87 = Unbundle(w398) -> ("Frequency out"=w397:dbl, "Resistance out"=w396:dbl)
          n88 = Bundle("arduino addresses out"=w385, w395, "Address out"=w394, w393, w392, "SRS address out"=w391) -> (w390:T26)  [unwired: 1 in]
        }
        n89 = call "turbo_pump_on_off 11-08-2017.vi"("Turbo pump\nauto on"=w257, "pressure control on?"=w315, "error in (no error)"=w330, "read pressure"=w313, "read pressure 2"=w314, "VISA Refnum in"=w331) -> ("error out"=w329:errorcluster, "VISA Refnum out"=w328:refnum<visa-resource-name>)  [unwired: 4 in]
        n90 = Boolean To (0,1)(Boolean=w339) -> (0, 1=w355:i16)
        n91 = Boolean To (0,1)(Boolean=w338) -> (0, 1=w354:i16)
        n92 = Equal To 0?(x=w355) -> (x = 0?=w352:bool)
        n93 = Not Equal To 0?(x=w354) -> (x != 0?=w353:bool)
        n94 = Unbundle By Name("SEQUENCE") -> ("Run Sequence"=w261:bool, "User-defined\nsequence"=w264:string[][], "preview"=w265:u16)
        n95 = And(x=w352, y=w353) -> (x .and. y?=w350:bool)
        n96 = And(x=w258, y=w350) -> (x .and. y?=w349:bool)
        n97 = Or(x=w349, y="Stop") -> (x .or. y?=w351:bool)
        n98 = call "Elapsed Time2"() -> ("Present (s)"=w279:dbl)  [unwired: 12 in, 7 out]
        n99 = Or(x=w259, y=w261) -> (x .or. y?=w252:bool)
        "saving data?" <- w252
        n100 = Bundle("User-defined\nsequence"=w264, "Present (s)"=w279, "current  step # in"=w337, "sequence end time in"=w340) -> (w344:T27)  [unwired: 1 in]
        n101 = call "plot_usr_seq_selectableDisplay.vi"("Display"=w265, "User-defined sequence"=w264) -> ("Sequence Preview"=w263:cluster{dbl[], dbl[]}[], "seq length (hours)"=w244:dbl)  [unwired: 8 in]
        n102 = call "Pressure_control_subVI _newturbo.vi"("Run Sequence"=w261, "user sequence, present (s) in, current step in, seq time in"=w344, "pressure parameters in"=w274, "pressure control on?/daq IDs/errors"=w332) -> ("current step # out, shift register time out, seq button on?"=w343:T28, "sequence over? USE THIS TO REINITIALIZE RUN SEQUENCE BUTTON SO PROGRAM ENDS"=w262:bool, "save press/RH/gasflow/vaporflow - read valve position/pressure/vaporflow/gasflow"=w335:T29, "pressure control on?/daq IDs/errors out"=w336:T30, "sequence end date/time string"=w255:string, "pressure_setpoint"=w333:string)  [unwired: 2 in]
        n103 = property on="Length (hrs)" class="DigNum (strict)"("Value"=w244) -> ()  [unwired: 2 in, 2 out]
        n104 = property on="Sequence\npreview" class="XYGraph (strict)"("Value"=w263) -> ()  [unwired: 2 in, 2 out]
        n105 = case shown="True" w262 {
          frame False {
          }
          frame True {
            n106 = property on="Run Sequence" class="Bool (strict)"("Value"=FALSE ("Run Sequence")) -> ()  [unwired: 2 in, 2 out]
          }
        }
        n107 = property on="End time" class="Str"("Value"=w255) -> ()  [unwired: 2 in, 2 out]
        n108 = Transpose 2D Array(2D array=w293) -> (transposed array=w292:dbl[][])
        n109 = call-poly <vilib>:"Mean.vi"("X"=w299) -> ("mean"=w297:dbl)  [unwired: 1 out]
        n110 = call-poly <vilib>:"Mean.vi"("X"=w298) -> ("mean"=w296:dbl)  [unwired: 1 out]
        n111 = call-poly <vilib>:"Mean.vi"("X"=w307) -> ("mean"=w309:dbl)  [unwired: 1 out]
        n112 = call-poly <vilib>:"Mean.vi"("X"=w302) -> ("mean"=w247:dbl)  [unwired: 1 out]
        "K-2420" <- w247
        n113 = for {
          tunnel: w292 -> [w383] mode=indexing
          tunnel: [w384] -> w291 mode=indexing
          # "average each signal and remove extreme outliers"
          n114 = call "remove_array_outliers 11-16-2017.vi"("n standard devs to filter"=2.5, "input array"=w383) -> ("filtered array out"=w382:dbl[])  [unwired: 9 in]
          n115 = call-poly <vilib>:"Mean.vi"("X"=w382) -> ("mean"=w384:dbl)  [unwired: 1 out]
        }
        n116 = call-poly <vilib>:"Mean.vi"("X"=w301) -> ("mean"=w246:dbl)  [unwired: 1 out]
        "K-2100" <- w246
        n117 = call-poly <vilib>:"Mean.vi"("X"=w305) -> ("mean"=w303:dbl)  [unwired: 1 out]
        "J-KEM temp" <- w303
        n118 = Bundle("mean"=w297, "mean"=w296) -> (w295:cluster{"mean":dbl, "mean":dbl})  [unwired: 1 in]
        "QCM plot" <- w295
        n119 = Number To Engineering String(2:w285, 3:w285, 4:w309) -> (0:w308:string)  [unwired: 1 in]
        n120 = Number To Engineering String(2:w283, 3:w283, 4:w247) -> (0:w306:string)  [unwired: 1 in]
        n121 = Unbundle(w335) -> ("press/RH/gas/vapor"=w334:T31, "Cluster"=w278:T32)
        n122 = Number To Engineering String(2:w282, 3:w282, 4:w246) -> (0:w300:string)  [unwired: 1 in]
        n123 = Number To Engineering String(2:w280, 3:w280, 4:w295) -> (0:w294:cluster{"mean":string, "mean":string})  [unwired: 1 in]
        n124 = Number To Engineering String(2:w284, 3:w284, 4:w303) -> (0:w304:string)  [unwired: 1 in]
        n125 = Unbundle(w278) -> ("Valve position (%)"=w277:dbl, "read pressure"=w256:dbl, "read vapor flow"=w276:dbl, "read gas flow"=w275:dbl)
        "pressure chart" <- w256
        n126 = Array To Cluster(array=w291) -> (cluster=w290:T4)
        "arduino qcm stack plot" <- w290
        n127 = property on="Actual" class="DigNum (strict)"("Value"=w277) -> ()  [unwired: 2 in, 2 out]
        n128 = property on="Read vapor flow (sccm)" class="DigNum (strict)"("Value"=w276) -> ()  [unwired: 2 in, 2 out]
        n129 = Number To Engineering String(2:w281, 3:w281, 4:w290) -> (0:w289:T33)  [unwired: 1 in]
        n130 = property on="Read gas flow (sccm)" class="DigNum (strict)"("Value"=w275) -> ()  [unwired: 2 in, 2 out]
        n131 = property on="Read pressure (Torr)" class="DigNum (strict)"("Value"=w256) -> ()  [unwired: 2 in, 2 out]
        n132 = call "Elapsed Time"() -> ("Elapsed Time (s)"=w310:dbl)  [unwired: 12 in, 7 out]
        n133 = event shown="[1] \"Clear all charts\": Value Change" {
          selector: _ -> [_ _ _ _ _]
          dyn-events: _ -> [_ _ _ _ _]
          timeout: 20 -> [_ _ _ _ _]
          event Timeout {
            n134 = event-data() -> ()  [unwired: 1 in, 1 out]
          }
          event "Clear all charts": Value Change {
            w375 = dbl[] [] ("History Data")
            n135 = event-data() -> ()  [unwired: 1 in, 1 out]
            n136 = property on="arduino qcm stack plot" class="WFChart (strict)"("History Data"=T10 []) -> ()  [unwired: 2 in, 2 out]
            n137 = property on="J-KEM temp" class="WFChart (strict)"("History Data"=w375) -> ()  [unwired: 2 in, 2 out]
            n138 = property on="pressure chart" class="WFChart (strict)"("History Data"=w375) -> ()  [unwired: 2 in, 2 out]
            n139 = property on="K-2420" class="WFChart (strict)"("History Data"=w375) -> ()  [unwired: 2 in, 2 out]
            n140 = property on="QCM plot" class="WFChart (strict)"("History Data"=T11 []) -> ()  [unwired: 2 in, 2 out]
            n141 = property on="K-6430" class="WFChart (strict)"("History Data"=w375) -> ()  [unwired: 2 in, 2 out]
          }
          event "SEQUENCE.Clear sequence": Value Change {
            n142 = event-data() -> ()  [unwired: 1 in, 1 out]
            n143 = property on="User-defined\nsequence" class="Tbl (strict)"("Value"=string[][] []) -> ()  [unwired: 2 in, 2 out]
          }
          event "SEQUENCE.Save sequence": Value Change {
            n144 = event-data() -> ()  [unwired: 1 in, 1 out]
            n145 = property on="User-defined\nsequence" class="Tbl (strict)"() -> ("Value"=w379:string[][])  [unwired: 2 in, 2 out]
            n146 = call-poly <vilib>:"Write To Spreadsheet File.vi"("2D data"=w379) -> ()  [unwired: 7 in, 1 out]
          }
          event "SEQUENCE.Import sequence file": Value Change {
            n147 = event-data() -> ()  [unwired: 1 in, 1 out]
            n148 = call-poly <vilib>:"Read From Spreadsheet File.vi"() -> ("all rows"=w380:string[][])  [unwired: 7 in, 4 out]
            n149 = property on="User-defined\nsequence" class="Tbl (strict)"("Value"=w380) -> ()  [unwired: 2 in, 2 out]
          }
        }
        n150 = Get Date/Time In Seconds() -> (seconds since 1Jan1904=w364:timestamp)
        n151 = expression code="x/60"(w310) -> (w311:dbl)
        n152 = Format Date/Time String(time format string (%c)="%Y-%m-%d %H:%M:%S%2u", seconds (now)=w364) -> (date/time string=w360:string)  [unwired: 1 in]
        n153 = Number To Engineering String ("elapsed time (min)")(4:w311) -> (0:w346:string)  [unwired: 3 in]
        n154 = Unbundle(w294) -> ("mean"=w347:string, "mean"=w361:string)
        n155 = Unbundle(w334) -> ("pressure"=w359:string, "RH"=w358:string, "gas flow"=w357:string, "vapor flow"=w356:string)
        n156 = Unbundle(w289) -> ("[0]"=w326:string, "[1]"=w325:string, "[2]"=w324:string, "[3]"=w323:string, "[4]"=w322:string, "[5]"=w321:string)
        n157 = Build Array(w360, w346, w304, w308, w306, w300, w347, w361, w359, w358, w357, w356, w333, w326, w325, w324, w323, w322, w321) -> (w254:string[])
        n158 = case shown="True" w252 {
          tunnel: w254 -> [_ w374]
          tunnel: [w365 w371] -> w253
          tunnel: w248 -> [w366 w370]
          frame False {
            # "Do not save data now"
            n159 = Unbundle(w366) -> (w365:string[][])  [unwired: 2 out]
          }
          frame True {
            # "Save data now"
            n160 = Unbundle(w370) -> (w369:string[][], w368:path, "data headers"=w367:string[])
            n161 = Build Array (concatenate)(w369, w374) -> (w371:string[][])
            n162 = call-poly <vilib>:"Write To Spreadsheet File.vi"("1D data"=w367, "file path (dialog if empty)"=w368) -> ("new file path (Not A Path if cancelled)"=w372:path)  [unwired: 6 in]
            n163 = call-poly <vilib>:"Write To Spreadsheet File.vi"("append to file? (new file:F)"=TRUE, "2D data"=w371, "file path (dialog if empty)"=w372) -> ()  [unwired: 5 in, 1 out]
          }
        }
        n164 = Unbundle(w343) -> ("current  step # in"=w312:i32, "sequence end time in"=w342:timestamp, "Boolean"=w341:bool)
        n165 = Index Array "current bias setpoint"(array=w264, index (row)=w312, index (col)=4 ("disabled index (col)")) -> ()  [unwired: 1 out]
        n166 = Increment(x=w312) -> ()  [unwired: 1 out]
        "State date/time" <- w345
      }
      n167 = Unbundle(w58) -> ("Boolean"=w57:bool, "task out"=w44:refnum<k21>, "error out"=w43:errorcluster, "task out"=w42:refnum<k21>, "error out"=w41:errorcluster, "VISA resource name out"=w40:refnum<visa-resource-name>, "error out"=w39:errorcluster)
      n168 = Unbundle(w19) -> ("arduino addresses out"=w18:T25, w17:T17, "Address out"=w16:T23, w15:T17, w14:T17, "SRS address out"=w13:T24)
      n169 = case shown="True" w57 {
        tunnel: [errorcluster {"status"=FALSE, "code"=0, "source"=""} ("error out") w118] -> w61
        tunnel: w44 -> [_ w117]
        tunnel: w43 -> [_ w116]
        tunnel: w42 -> [_ w115]
        tunnel: w41 -> [_ w112]
        tunnel: w40 -> [_ w113]
        tunnel: w39 -> [_ w114]
        tunnel: w35 -> [_ w109]
        tunnel: w34 -> [_ w108]
        frame False {
          # "Pressure control close"
        }
        frame True {
          # "Pressure control close"
          n170 = call <vilib>:"DAQmx Stop Task.vi"("task/channels in"=w117, "error in"=w116) -> ("task out"=w124:refnum<k21>, "error out"=w123:errorcluster)  [unwired: 12 in]
          n171 = call <vilib>:"DAQmx Stop Task.vi"("task/channels in"=w115, "error in"=w112) -> ("task out"=w125:refnum<k21>, "error out"=w126:errorcluster)  [unwired: 12 in]
          n172 = VISA Clear(VISA resource name=w113, error in (no error)=w114) -> (VISA resource name out=w122:refnum<visa-resource-name>, error out=w121:errorcluster)
          n173 = VISA Close(VISA resource name=w109, error in (no error)=w108) -> (error out=w110:errorcluster)
          n174 = VISA Close(VISA resource name=w122, error in (no error)=w121) -> (error out=w111:errorcluster)
          n175 = call <vilib>:"DAQmx Clear Task.vi"("task in"=w124, "error in"=w123) -> ("error out"=w120:errorcluster)  [unwired: 13 in]
          n176 = call <vilib>:"DAQmx Clear Task.vi"("task in"=w125, "error in"=w126) -> ("error out"=w119:errorcluster)  [unwired: 13 in]
          n177 = Merge Errors(w120, w119, w111, w110) -> (w118:errorcluster)
        }
      }
      n178 = Unbundle(w13) -> ("Boolean"=w77:bool, "VISA out"=w76:refnum<visa-resource-name>, "error out"=w22:errorcluster)
      n179 = Unbundle(w15) -> (w80:bool, "VISA resource name out"=w79:refnum<visa-resource-name>, "error out"=w78:errorcluster)
      n180 = Unbundle(w14) -> (w25:bool, "VISA resource name out"=w24:refnum<visa-resource-name>, "error out"=w23:errorcluster)
      n181 = Unbundle(w17) -> (w70:bool, "VISA resource name out"=w69:refnum<visa-resource-name>, "error out"=w68:errorcluster)
      n182 = call "arduino_close_subIV 11-08-2017.vi"("arduino addresses out"=w18) -> ()  [unwired: 11 in]
      n183 = Unbundle(w16) -> ("Boolean"=w74:bool, "VISA resource name out"=w73:refnum<visa-resource-name>, "error out"=w72:errorcluster)
      n184 = case shown="False" w77 {
        tunnel: [w200 w203] -> w21
        tunnel: w76 -> [_ w202]
        tunnel: w22 -> [w200 w201]
        frame False {
          # "SRS-200 close"
        }
        frame True {
          # "SRS-200 close"
          n185 = call "srsQcm200Close.vi"("error in"=w201, "Visa in"=w202) -> ("error out"=w203:errorcluster)  [unwired: 3 in]
        }
      }
      n186 = case shown="True" w25 {
        tunnel: w24 -> [_ w91]
        tunnel: w23 -> [w88 w90]
        tunnel: [w88 w89] -> w64
        frame False {
          # "Keithley-2100 close"
        }
        frame True {
          # "Keithley-2100 close"
          n187 = call "Close.vi"("VISA resource name"=w91, "error in (no error)"=w90) -> ("error out"=w89:errorcluster)  [unwired: 17 in]
        }
      }
      n188 = case shown="True" w80 {
        tunnel: w79 -> [_ w219]
        tunnel: w78 -> [w216 w218]
        tunnel: [w216 w217] -> w81
        frame False {
          # "Keithley-2420 close"
        }
        frame True {
          # "Keithley-2420 close"
          n189 = call "Enable Output.vi"("error in (no error)"=w218, "Enable Output (T: Enable)"=FALSE, "VISA resource name"=w219) -> ("error out"=w220:errorcluster, "VISA resource name out"=w222:refnum<visa-resource-name>)  [unwired: 7 in]
          n190 = call "Close.vi"("error in (no error)"=w220, "VISA resource name"=w222) -> ("error out"=w217:errorcluster)  [unwired: 9 in]
        }
      }
      n191 = case shown="True" w70 {
        tunnel: w69 -> [_ w157]
        tunnel: w68 -> [w155 w156]
        tunnel: [w155 w158] -> w67
        frame False {
          # "Keithley-6430 close"
        }
        frame True {
          # "Keithley-6430 close"
          n192 = call "Enable Output.vi"("error in (no error)"=w156, "Enable Output (F:Off)"=FALSE ("Output (F:Off)"), "VISA resource name"=w157) -> ("error out"=w159:errorcluster, "VISA resource name out"=w160:refnum<visa-resource-name>)  [unwired: 7 out]
          n193 = call "Close.vi"("error in (no error)"=w159, "VISA resource name"=w160) -> ("error out"=w158:errorcluster)  [unwired: 9 out]
        }
      }
      n194 = case shown="True" w74 {
        tunnel: w73 -> [_ w188]
        tunnel: w72 -> [w185 w187]
        tunnel: [w185 w186] -> w71
        frame False {
          # "J-KEM close"
        }
        frame True {
          # "J-KEM close"
          n195 = VISA Close(VISA resource name=w188, error in (no error)=w187) -> (error out=w186:errorcluster)
        }
      }
      n196 = call <vilib>:"Simple Error Handler.vi"("error in (no error)"=w61) -> ()  [unwired: 4 in, 5 out]
      n197 = flat-sequence {
        tunnel: w21 -> [w87]
        tunnel: [w87] -> w20
        frame #0 {
          w86 = FALSE ("saving data?")
          # "re-initialize settings"
          n198 = property on="saving data?" class="Bool (strict)"("Value"=w86) -> ()  [unwired: 2 in, 2 out]
          n199 = property on="Run Sequence" class="Bool (strict)"("Value"=w86) -> ()  [unwired: 2 in, 2 out]
        }
      }
      n200 = Merge Errors(w67, w71, w81, w64, w20) -> (w82:errorcluster)
      n201 = call <vilib>:"Simple Error Handler.vi"("error in (no error)"=w82) -> ()  [unwired: 4 in, 5 out]
    }
  }
